vi "Encrypt.vi"(11 "Letter in":refnum<class "Letter.lvclass">) -> (2 "letter":string, 3 "Letter out":refnum<class "Letter.lvclass">)   [LabVIEW 2015, in "Letter.lvclass"]
uses:
  Letter.lvclass
  Letter.lvclass/Letter.ctl
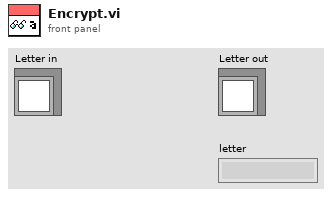
[diagram p1: front panel]
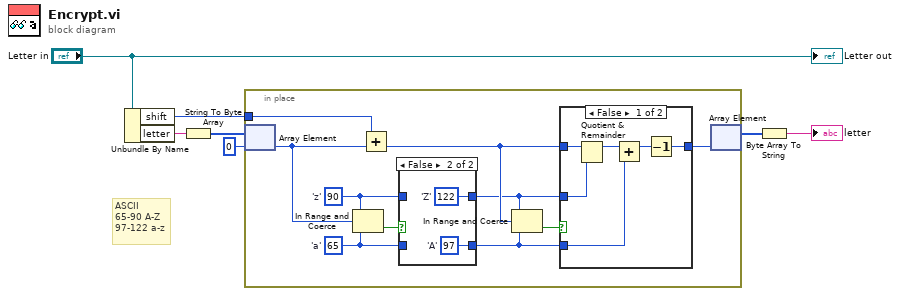
[diagram p0: block diagram]
diagram:
  # "ASCII\n65-90 A-Z\n97-122 a-z"
  n1 = Unbundle By Name("Letter in") -> ("shift"=w1:u8, "letter"=w6:string)
  n2 = String To Byte Array(string=w6) -> (unsigned byte array=w4:u8[])
  n3 = in-place {
    in-place-border: w1 -> [w17]
    w13 = u8 90  # 'z'
    w12 = u8 65  # 'a'
    n4 = in-place-array #1(w4, 0) -> (w16:u8)
    n5 = In Range and Coerce(upper limit=w13, x=w16, lower limit=w12) -> (In Range?=w14:bool)  [unwired: 1 out]
    n6 = Add(x=w17, y=w16) -> (x+y=w11:u8)
    n7 = case shown="False" w14 {
      tunnel: w13 -> [w26 _]
      tunnel: w12 -> [w25 _]
      tunnel: [w26 w28] -> w10
      tunnel: [w25 w27] -> w8
      frame True {
      }
      frame False {
        w28 = u8 122  # 'Z'
        w27 = u8 97  # 'A'
      }
    }
    n8 = In Range and Coerce(upper limit=w10, x=w11, lower limit=w8) -> (In Range?=w9:bool)  [unwired: 1 out]
    n9 = case shown="False" w9 {
      tunnel: [w18 w24] -> w15
      tunnel: w11 -> [w21 w24]
      tunnel: w10 -> [w20 _]
      tunnel: w8 -> [w19 _]
      frame False {
        n10 = Quotient & Remainder(x=w21, y=w20) -> (x-y*floor(x/y)=w23:u8)  [unwired: 1 out]
        n11 = Add(x=w23, y=w19) -> (x+y=w22:u8)
        n12 = Decrement(x=w22) -> (x-1=w18:u8)
      }
      frame True {
      }
    }
    n13 = in-place-array #1(w15) -> (w3:u8[])  [unwired: 1 out]
  }
  n14 = Byte Array To String(unsigned byte array=w3) -> (string=→"letter":string)
  "Letter out" <- "Letter in"
